vi "Configure Sequencer List All Signals.vi"(6 "Signals (\"'CW','CW'\")":string="'CW','CW'", 8 "error in (no error)":errorcluster, 10 "Instance (1)":i32=1, 11 "VISA resource name":refnum<visa-resource-name>) -> (0 "error out":errorcluster, 3 "VISA resource name out":refnum<visa-resource-name>)   [LabVIEW 2020, in "Rohde&Schwarz CMXP GPRF.lvlib"]
doc: "Defines the signal types for all sequencer list entries.\n\nAttribute:\nRSCMXPGPRF_ATTR_SEQUENCER_LIST_ALL_SIGNALS\n\nRemote-control command:\nSOURce:GPRF:GEN<i>:SEQuencer:LIST:SIGNal:ALL"
uses:
  <instrlib>/Rohde&Schwarz CMXP GPRF/Rohde&Schwarz CMXP GPRF.lvlib
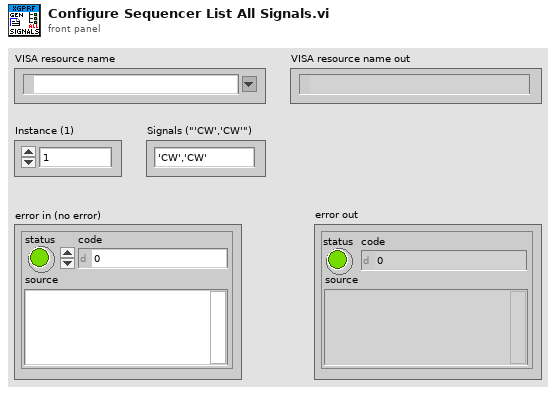
[diagram p1: front panel]
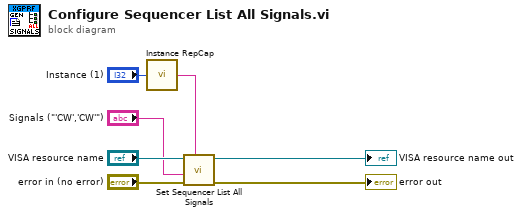
[diagram p0: block diagram]
diagram:
  n1 = call <instrlib>:"Instance RepCap.vi"("Instance in"="Instance (1)") -> ("Instance out"=w2:string)
  n2 = call "Set Sequencer List All Signals"("Repeated Capabilities"=w2, "error in (no error)"="error in (no error)", "Sequencer List All Signals ()"="Signals (\"'CW','CW'\")", "instrument handle"="VISA resource name") -> ("error out"=→"error out":errorcluster, "instrument handle out"=→"VISA resource name out":refnum<visa-resource-name>)  [unwired: 6 in]
